vi "Override Joystick.vi"() -> ()   [LabVIEW 2011]
uses:
  <vilib>/Rock Robotics/WPI/Joystick/WPI_JoystickDeviceEnum.ctl
  <vilib>/Rock Robotics/WPI/Joystick/WPI_JoystickDevRef.ctl
panel:
  in  "JoystickDevRef":T1
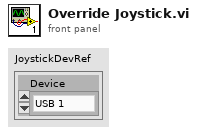
[diagram p1: front panel]
types:
  T1 = typedef "WPI_JoystickDevRef.ctl" = cluster{"Device":T2}
  T2 = typedef "WPI_JoystickDeviceEnum.ctl" = enum16{"USB 1", "USB 2", "USB 3", "USB 4", "Kinect 1", "Kinect 2"}
  T3 = typedef "WPI_JoystickButtonState.ctl" = cluster{"Button 1":bool, "Button 2":bool, "Button 3":bool, "Button 4":bool, "Button 5":bool, "Button 6":bool, "Button 7":bool, "Button 8":bool, "Button 9":bool, "Button 10":bool, "Button 11":bool, "Button 12":bool}
  T4 = cluster{"axis 1 (x)":dbl, "axis 2 (y)":dbl, "axis 3 (throttle)":dbl, "axis 4":dbl, "axis 5":dbl, "axis 6":dbl}
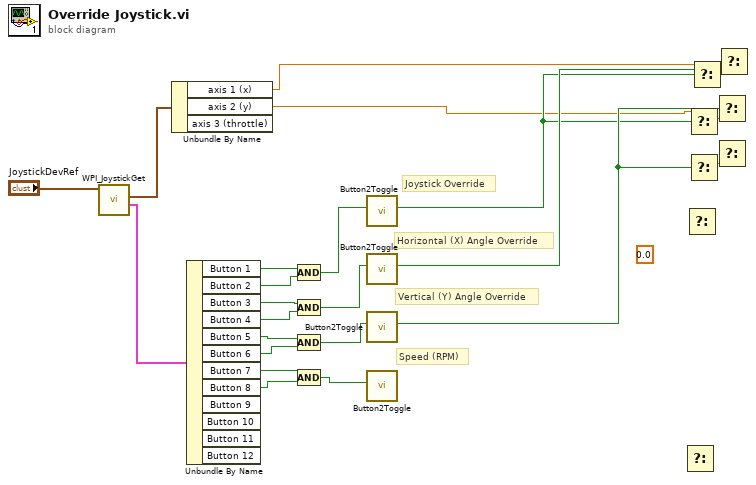
[diagram p0: block diagram]
diagram:
  (unwired) 0.0 ("f")
  # "Joystick Override"
  # "Speed (RPM)"
  # "Vertical (Y) Angle Override"
  # "Horizontal (X) Angle Override"
  n1 = call <vilib>:"WPI_JoystickGet.vi"("JoystickDevRef"="JoystickDevRef") -> ("Buttons"=w21:T3, "Axes"=w22:T4)  [unwired: 4 in, 1 out]
  n2 = Unbundle By Name(w22) -> ("axis 1 (x)"=w8:dbl, "axis 2 (y)"=w1:dbl)  [unwired: 1 out]
  n3 = Unbundle By Name(w21) -> ("Button 1"=w20:bool, "Button 2"=w19:bool, "Button 3"=w17:bool, "Button 4"=w16:bool, "Button 5"=w18:bool, "Button 6"=w15:bool, "Button 7"=w14:bool, "Button 8"=w13:bool)  [unwired: 4 out]
  n4 = Compound Arithmetic op=AND(w20, w19) -> (w12:bool)
  n5 = Compound Arithmetic op=AND(w17, w16) -> (w11:bool)
  n6 = Compound Arithmetic op=AND(w18, w15) -> (w10:bool)
  n7 = Compound Arithmetic op=AND(w14, w13) -> (w9:bool)
  n8 = call "Button2Toggle.vi"("Boolean"=w12) -> ("Latched Boolean"=w2:bool)  [unwired: 9 in, 1 out]
  n9 = call "Button2Toggle.vi"("Boolean"=w11) -> ("Latched Boolean"=w4:bool)  [unwired: 9 in, 1 out]
  n10 = call "Button2Toggle.vi"("Boolean"=w10) -> ("Latched Boolean"=w3:bool)  [unwired: 9 in, 1 out]
  n11 = call "Button2Toggle.vi"("Boolean"=w9) -> ()  [unwired: 9 in, 2 out]
  n12 = Select() -> ()  [unwired: 3 in, 1 out]
  n13 = Select() -> ()  [unwired: 3 in, 1 out]
  n14 = Select(t=w1, s=w2) -> (s? t:f=w6:dbl)  [unwired: 1 in]
  n15 = Select(s=w3) -> (s? t:f=w5:dbl)  [unwired: 2 in]
  n16 = Select(t=w8, s=w2) -> (s? t:f=w7:dbl)  [unwired: 1 in]
  n17 = Select(s=w3, f=w6) -> ()  [unwired: 1 in, 1 out]
  n18 = Select(f=w5) -> ()  [unwired: 2 in, 1 out]
  n19 = Select(s=w4, f=w7) -> ()  [unwired: 1 in, 1 out]
